vi "svl_Log View for Peak Resampled Level (N Ch) (single value).vi"(7 "even angle channel info":T1[](array[typedef]) {"channel info"."pregain" format="%.2f"; "channel info"."weighting filter" items=["Linear", "A-weighting", "B-weighting", "C-weighting", "ITU-R 468-4", "Dolby", "CCITT", "C-message", "Wb", "Wc", "Wd", "We", "Wf", "Wh", "Wj", "Wk", "Wm", "AES17 20 kHz lowpass", "AES17 40 kHz lowpass", "AES17 20 kHz highpass", "AES17 40 kHz highpass"]; "channel info"."dB reference" format="%^.1e"; "channel info"."engineering units" items=["custom..."=0, "V"=1, "A"=21, "C"=30, "pC"=31, "s"=32, "-"=29, "Pa"=2, "N"=20, "g"=3, "m/s^2"=4, "m/s"=5, "m"=6, "mm/s"=12, "mm"=13, "micron/s"=14, "micron"=15, "in/s^2"=7, "in/s"=8, "in"=9, "mil/s"=10, "mil"=11, "rad/s^2"=16, "rad/s"=17, "rad"=18, "deg/s^2"=26, "deg/s"=27, "deg"=28, "RPM"=22, "cycle/s^2"=23, "Hz"=24, "cycle"=25, "strain"=19]; "channel info"."sensor sensitivity" format="%#_5f"}, 8 "error in (no error)":errorcluster, 10 "dB On (T)":bool=TRUE, 11 "peak levels [EU]":dbl[](array[numeric]) format="%.2f") -> (0 "error out":errorcluster, 2 "unit label [ ]":string[](array[string]), 3 "peak levels [EU]":dbl[](array[numeric]) format="%.2f")   [LabVIEW 2017]
uses:
  <vilib>/addons/_NISVFA/_Shared subVIs/Controls/svc_Resampled Channel Info.ctl
  <vilib>/addons/_NISVFA/_Shared subVIs/Controls/svc_Channel Info.ctl
  <vilib>/addons/_NISVFA/_Shared subVIs/Controls/svc_Engineering Units Text Ring.ctl
  <vilib>/addons/_NISVFA/_Shared subVIs/Controls/svc_Weighting Filter Text Ring.ctl
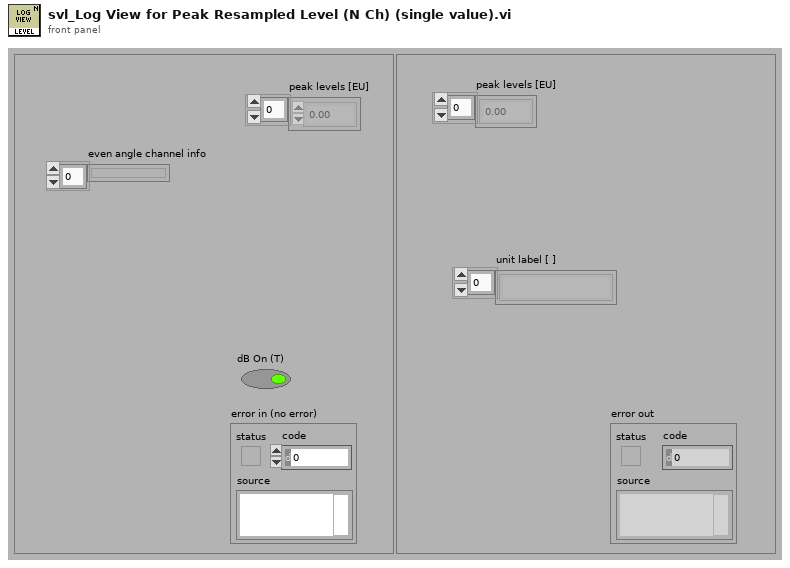
[diagram p1: front panel]
types:
  T1 = typedef "svc_Resampled Channel Info.ctl" = cluster{"channel name":string, "description":string, " channel info":T2}
  T2 = typedef "svc_Channel Info.ctl" = cluster{"sensor sensitivity":dbl, "engineering units":T3, "dB reference":dbl, "custom label":string, "weighting filter":T4, "pregain":dbl}
  T3 = typedef "svc_Engineering Units Text Ring.ctl" = u16
  T4 = typedef "svc_Weighting Filter Text Ring.ctl" = u16
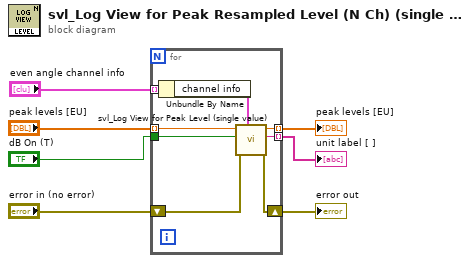
[diagram p0: block diagram]
diagram:
  n1 = for {
    tunnel: "peak levels [EU]" -> [w14] mode=indexing
    tunnel: "dB On (T)" -> [w12]
    tunnel: "even angle channel info" -> [w10] mode=indexing
    tunnel: [w13] -> w6 mode=indexing
    tunnel: [w11] -> w5 mode=indexing
    shift-right: [w15] -> w2
    shift-left: "error in (no error)" -> [w9]
    n2 = Unbundle By Name(w10) -> ("channel info"=w8:T2)
    n3 = call <vilib>:"svl_Log View for Peak Level (single value).vi"("channel info"=w8, "error in (no error)"=w9, "dB On (T)"=w12, "peak level [EU]"=w14) -> ("error out"=w15:errorcluster, "unit label"=w11:string, "peak level [EU]"=w13:dbl)  [unwired: 5 in]
  }
  "unit label [ ]" <- w5
  "peak levels [EU]" <- w6
  "error out" <- w2
